vi "write controls values.vi"(6 "call chain index (1)":i32=1, 7 "vi ref (caller)":refnum<vi>, 8 "error in (no error)":errorcluster, 10 "values":variant[](array[variant]), 11 "labels":string[](array[string])) -> (0 "error out":errorcluster)   [LabVIEW 2024, in "controls manager.lvlib"]
uses:
  controls manager.lvlib
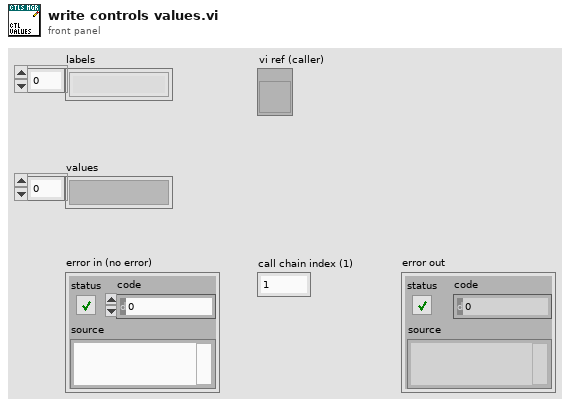
[diagram p1: front panel]
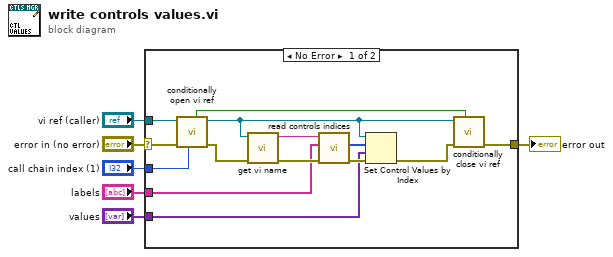
[diagram p0: block diagram]
diagram:
  n1 = case shown="No Error" "error in (no error)" {
    selector: "error in (no error)" -> [w19 w21]
    tunnel: [w16 w21] -> w6
    tunnel: "vi ref (caller)" -> [w13 _]
    tunnel: "call chain index (1)" -> [w12 _]
    tunnel: "labels" -> [w9 _]
    tunnel: "values" -> [w7 _]
    frame No Error {
      n2 = call "conditionally open vi ref.vi"("call chain index (1)"=w12, "error in (no error)"=w19, "vi ref in"=w13) -> ("error out"=w18:errorcluster, "vi ref out"=w10:refnum<vi>, "new ref?"=w15:bool)  [unwired: 6 in]
      n3 = call "get vi name.vi"("error in (no error)"=w18, "vi ref"=w10) -> ("error out"=w20:errorcluster, "vi name"=w14:string)  [unwired: 8 in]
      n4 = call "read controls indices.vi"("error in (no error)"=w20, "labels"=w9, "id"=w14) -> ("error out"=w17:errorcluster, "indices"=w11:i32[])  [unwired: 7 in]
      n5 = Set Control Values by Index(0:w10, 1:w11, 2:w7, 3:w17) -> (11:w8:errorcluster)
      n6 = call "conditionally close vi ref.vi"("new ref?"=w15, "error in (no error)"=w8, "vi ref"=w10) -> ("error out"=w16:errorcluster)  [unwired: 8 in]
    }
    frame Error {
    }
  }
  "error out" <- w6
